vi "[FPGA] SAR Acq Main.vi"() -> ()   [LabVIEW 2015]
doc: "This VI provides a template for customizing a waveform acquisition using scanned (or SAR) based NI C Series analog input modules."
uses:
  <vilib>/rvi/Emulation/niFpgaGetClockAttributes.vi
  <vilib>/rvi/Emulation/niFpgaSctlEmulationGetInTimedLoop.vi
  <vilib>/rvi/Emulation/niFpgaEmulationReportErrorSimple.vi
  <vilib>/rvi/Emulation/niFpgaProcessEmulError.vi
  <vilib>/rvi/interface/RandomDataEmulation/niFpgaRandomDataHandleErrors.vi
  <vilib>/rvi/eio/common/nirviEmuTemplateMethod_errors.vi
  <vilib>/rvi/Emulation/niFpgaCriticalErrorInLSC.vi
  <vilib>/rvi/DataTransferAndStorage/Container/XNode/niFpgaContainer.xnode
  <vilib>/rvi/interface/RandomDataEmulation/nirviRandomDataFpgaReadWriteTemplate.vi
  <vilib>/eio/EIONode/EIONode.xnode
panel:
  out "oclk freq":u32
  out "oclk div":u32
  out "oclk mult":u32
  in  "data rate (S/s)":u32
  in  "Chan Scale Array":sgl[](array[numeric])=[0.0, 0.0, 0.0, 0.0, 0.0, 0.0, 0.0, 0.0, 0.0, 0.0, 0.0, 0.0, 0.0, 0.0, 0.0, 0.0, 0.0, 0.0, 0.0, 0.0, 0.0, 0.0, 0.0, 0.0, 0.0, 0.0, 0.0, 0.0, 0.0, 0.0, 0.0, 0.0, 0.0, 0.0, 0.0, 0.0, 0.0, 0.0, 0.0, 0.0]
  out "Chan Count":bool
  out "Acq Loop Ticks":u32
  out "FPGA Error":errorcluster
  out "Module Underflow":bool
  out "Finished":bool
  in  "Number of Channels":i32=4
  in  "Samps per Chan [Finite]":i32=5120
  out "First Read":bool
  in  "Acquisition Type":enum16{"Finite Samples", "Continuous Samples"}(ring)
  out "DMA FIFO Full":bool
  in  "stop":bool
  # "Array size fixed at 40\nelements but may be \nexpanded if needed"
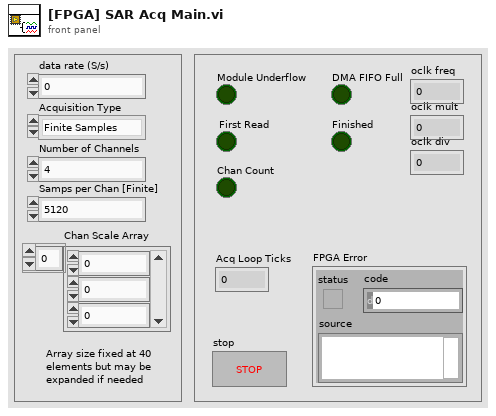
[diagram p1: front panel]
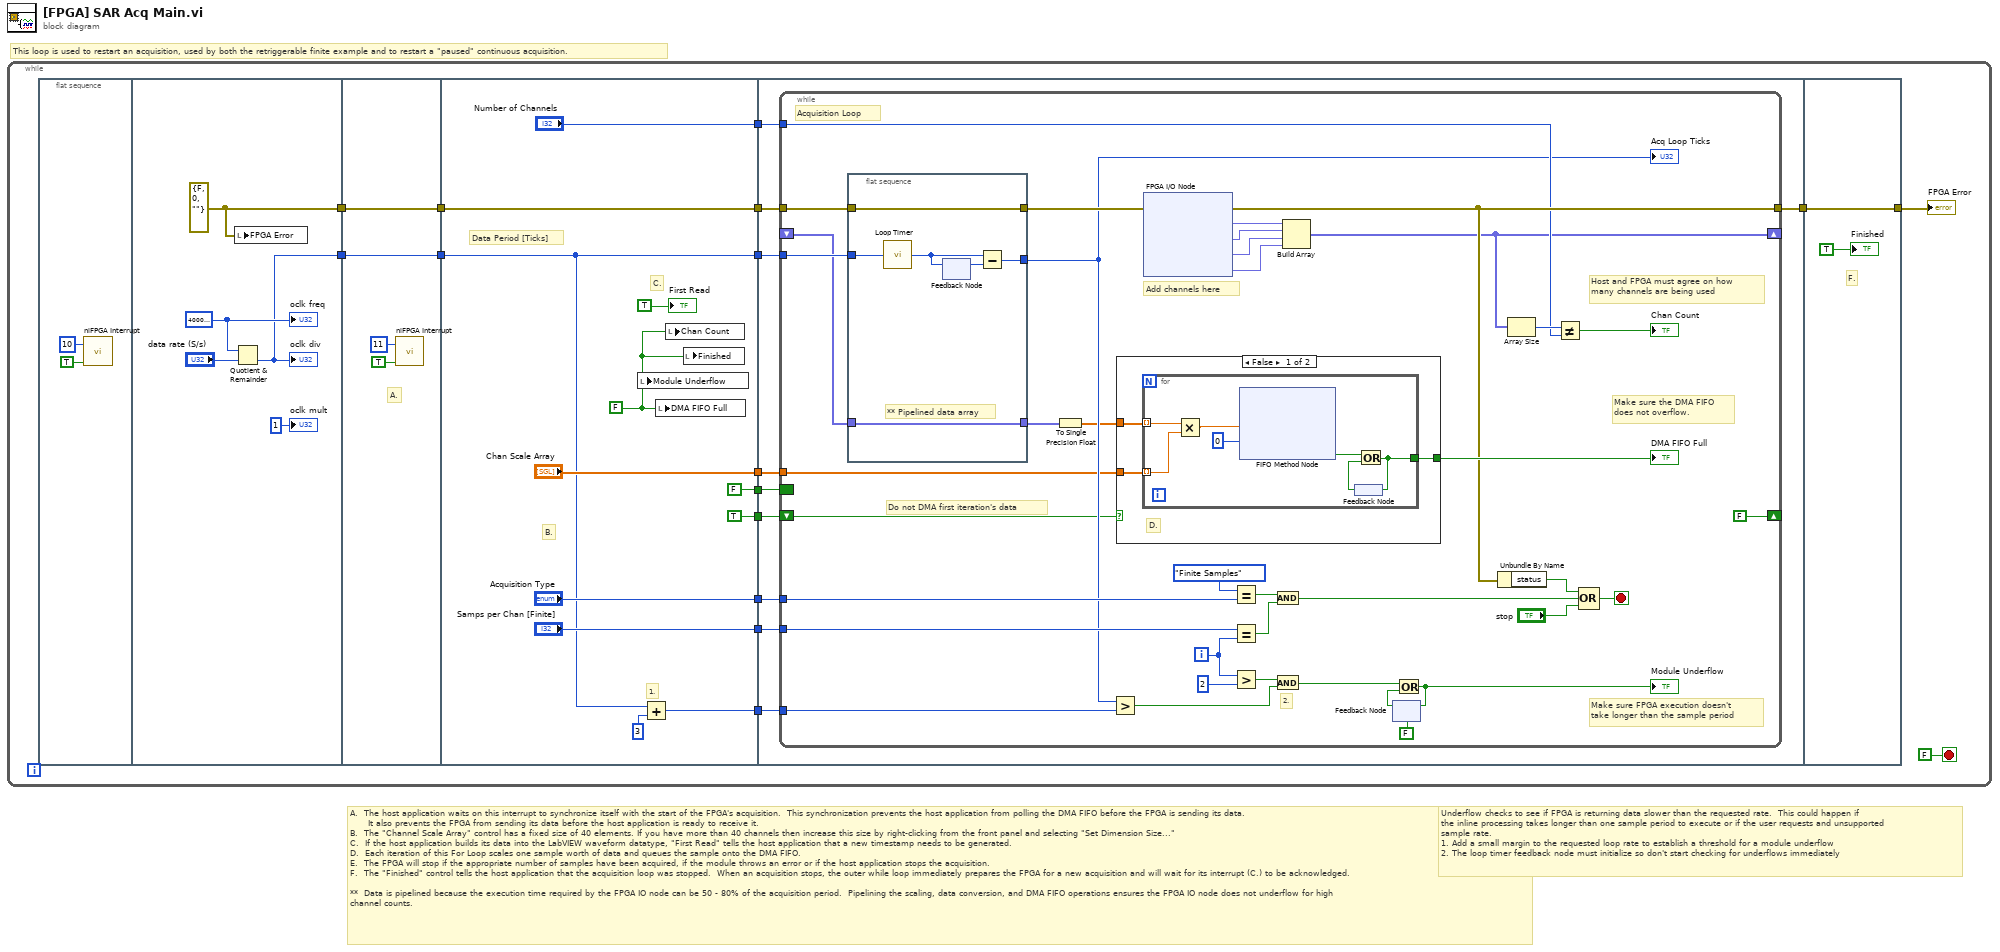
[diagram p0: block diagram]
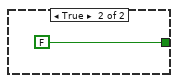
[diagram p2: hidden frame]
diagram:
  # "Underflow checks to see if FPGA is returning data slower than the requested rate.  This could happen if\nthe inline processing takes longer than one sample period to execute or if the user requests and unsupported\nsample rate.\n1. Add a small margin to the requested loop rate to establish a threshold for a module underflow \n2. The loop timer feedback node must initialize so don't start checking for underflows immediately"
  # "A.  The host application waits on this interrupt to synchronize itself with the start of the FPGA's acquisition.  This synchronization prevents the host application from polling the DMA FIFO before the FPGA is sending its data.\n      It also prevents the FPGA from sending its data before the host application is ready to receive it.\nB.  The \"Channel Scale Array\" control has a fixed size of 40 elements. If you have more than 40 channels then increase this size by right-clicking from the front panel and selecting \"Set Dimension Size...\"\nC.  If the host application builds its data into the LabVIEW waveform datatype, \"First Read\" tells the host application that a new timestamp needs to be generated.\nD.  Each iteration of this For Loop scales one sample worth of data and queues the sample onto the DMA FIFO.  \nE.  The FPGA will stop if the appropriate number of samples have been acquired, if the module throws an error or if the host application stops the acquisition.  \nF.  The \"Finished\" control tells the host application that the acquisition loop was stopped.  When an acquisition stops, the outer while loop immediately prepares the FPGA for a new acquisition and will wait for its interrupt (C.) to be acknowledged. \n\n**  Data is pipelined because the execution time required by the FPGA IO node can be 50 - 80% of the acquisition period.  Pipelining the scaling, data conversion, and DMA FIFO operations ensures the FPGA IO node does not underflow for high\nchannel counts."
  # "This loop is used to restart an acquisition, used by both the retriggerable finite example and to restart a \"paused\" continuous acquisition."
  n1 = while {
    stop <- FALSE stop-if-true
    n2 = flat-sequence {
      tunnel: [w20] -> w7
      tunnel: [w19] -> w3
      tunnel: w7 -> [w25]
      tunnel: [w25] -> w6
      tunnel: [w24] -> w4
      tunnel: w3 -> [w24]
      tunnel: ["Number of Channels"] -> w16
      tunnel: ["Chan Scale Array"] -> w15
      tunnel: ["Acquisition Type"] -> w14
      tunnel: ["Samps per Chan [Finite]"] -> w13
      tunnel: [w29] -> w12
      tunnel: [w33] -> w11
      tunnel: [TRUE] -> w10
      tunnel: w6 -> [w30]
      tunnel: [w30] -> w5
      tunnel: w4 -> [w29]
      tunnel: [FALSE] -> w2
      tunnel: w16 -> [w49]
      tunnel: w15 -> [w46]
      tunnel: w14 -> [w45]
      tunnel: w13 -> [w44]
      tunnel: w12 -> [w47]
      tunnel: w11 -> [w43]
      tunnel: w10 -> [w42]
      tunnel: [w41] -> w8
      tunnel: w5 -> [w48]
      tunnel: w2 -> [w40]
      tunnel: [w105] -> w9
      tunnel: w8 -> [w105]
      frame #0 {
        n3 = call <vilib>:"niFPGA Interrupt.vi"("Wait Until Cleared (F)"=TRUE ("Wait Until Cleared"), "IRQ Number (0)"=u8 10 ("IRQ Number")) -> ()  [unwired: 1 in]
      }
      frame #1 {
        w20 = errorcluster {"status"=FALSE, "code"=0, "source"=""} ("FPGA Error")
        w21 = u32 40000000 ("oclk freq")
        n4 = Quotient & Remainder(x=w21, y="data rate (S/s)") -> (floor(x/y)=w19:u32)  [unwired: 1 out]
        "oclk div" <- w19
        n5 = local write "FPGA Error"(w20) -> ()
        "oclk mult" <- u32 1 ("oclk mult")
        "oclk freq" <- w21
      }
      frame #2 {
        # "A."
        n6 = call <vilib>:"niFPGA Interrupt.vi"("Wait Until Cleared (F)"=TRUE ("Wait Until Cleared"), "IRQ Number (0)"=u8 11 ("IRQ Number")) -> ()  [unwired: 1 in]
      }
      frame #3 {
        w38 = FALSE ("Module Underflow")
        # "Data Period [Ticks]"
        # "1."
        # "C."
        # "B."
        n7 = local write "Module Underflow"(w38) -> ()
        n8 = Add(x=w29, y=u32 3) -> (x+y=w33:u32)
        n9 = local write "DMA FIFO Full"(w38) -> ()
        n10 = local write "Chan Count"(w38) -> ()
        n11 = local write "Finished"(w38) -> ()
        "First Read" <- TRUE ("First Read")
      }
      frame #4 {
        n12 = while {
          tunnel: w45 -> [w79]
          tunnel: w44 -> [w78]
          shift-right: [w52] -> _
          shift-left: _ -> [w65]
          tunnel: w49 -> [w80]
          tunnel: w48 -> [w67]
          tunnel: [w81] -> w41
          tunnel: w47 -> [w76]
          tunnel: w43 -> [w72]
          tunnel: w46 -> [w64]
          shift-right: [FALSE] -> _
          shift-left: w42 -> [w63]
          border: w40 -> [_]
          i -> [w61]
          stop <- w85 stop-if-true
          # "Add channels here"
          # "2."
          # "Do not DMA first iteration's data"
          # "Host and FPGA must agree on how \nmany channels are being used"
          # "Acquisition Loop"
          # "Make sure the DMA FIFO\ndoes not overflow."
          # "Make sure FPGA execution doesn't\ntake longer than the sample period"
          n13 = flat-sequence {
            tunnel: w76 -> [w103]
            tunnel: [w104] -> w77
            tunnel: w67 -> [w104]
            tunnel: [w100] -> w66
            tunnel: [w99] -> w51
            tunnel: w65 -> [w99]
            frame #0 {
              # "** Pipelined data array"
              n14 = call "Loop Timer"("Count(Ticks)"=w103) -> ("Tick Count(Ticks)"=w101:u32)
              n15 = feedback-in #1(w101) -> ()
              n16 = feedback #1() -> (w102:u32)  [unwired: 1 out]
              n17 = Subtract(x=w101, y=w102) -> (x-y=w100:u32)
            }
          }
          n18 = To Single Precision Float(number=w51) -> (single precision float=w50:sgl[])
          n19 = Greater?(x=w66, y=w72) -> (0:w75:bool)
          n20 = case shown="False" w63 {
            tunnel: [w90 FALSE] -> w84
            tunnel: w50 -> [w89 _]
            tunnel: w64 -> [w88 _]
            frame False {
              # "D."
              n21 = for {
                tunnel: [w96] -> w90
                tunnel: w89 -> [w95] mode=indexing
                tunnel: w88 -> [w94] mode=indexing
                n22 = Multiply(x=w95, y=w94) -> (x*y=w91:sgl)
                n23 = xnode ("FIFO Method Node")("Element"=w91, "Timeout"=0) -> ("Timed Out?"=w92:bool)  [unwired: 1 in, 1 out]
                n24 = feedback #2() -> (w97:bool)
                n25 = Or(x=w92, y=w97) -> (x .or. y?=w96:bool)
                n26 = feedback-in #2(w96) -> ()
              }
            }
            frame True {
            }
          }
          "DMA FIFO Full" <- w84
          n27 = xnode "FPGA I/O Node"("error in"=w77) -> ("error out"=w81:errorcluster, "Mod2/AI0"=w71:fxp<+/-,16,5>, "Mod2/AI1"=w70:fxp<+/-,16,5>, "Mod2/AI2"=w69:fxp<+/-,16,5>, "Mod2/AI3"=w68:fxp<+/-,16,5>)  [unwired: 4 in, 4 out]
          n28 = Equal?(x=enum16{"Finite Samples", "Continuous Samples"}."Finite Samples" ("y"), y=w79) -> (x = y?=w55:bool)
          n29 = Equal?(x=w78, y=w61) -> (x = y?=w54:bool)
          n30 = Greater?(x=w61, y=2) -> (0:w74:bool)
          n31 = And(x=w55, y=w54) -> (x .and. y?=w53:bool)
          n32 = And(x=w74, y=w75) -> (x .and. y?=w57:bool)
          n33 = Build Array(w71, w70, w69, w68) -> (w52:fxp<+/-,16,5>[])
          n34 = feedback #3(FALSE) -> (w59:bool)
          n35 = Or(x=w57, y=w59) -> (x .or. y?=w56:bool)
          "Module Underflow" <- w56
          n36 = feedback-in #3(w56) -> ()
          n37 = Unbundle By Name(w81) -> ("status"=w60:bool)
          n38 = Array Size(array=w52) -> (size(s)=w83:i32)
          n39 = Not Equal?(x=w83, y=w80) -> (x != y?=→"Chan Count":bool)
          n40 = Compound Arithmetic op=OR(w60, w53, "stop") -> (w85:bool)
          "Acq Loop Ticks" <- w66
        }
      }
      frame #5 {
        # "F."
        "Finished" <- TRUE ("Finished")
      }
    }
    "FPGA Error" <- w9
  }
